vi "add scan current(SubVI).vi"(10 "字符串":string) -> (1 "ok or cancel":bool=TRUE, 2 "连接的字符串":string)   [LabVIEW 2019, in "SubVI.lvlib"]
uses:
  SubVI.lvlib
panel:
  in  "Number of Step":i32=2
  in  "Increments (mA)":dbl=10.0
  in  "Final Current (mA)":dbl
  in  "Initial Current(mA)":dbl
  in  "cancel":bool
  in  "ok":bool
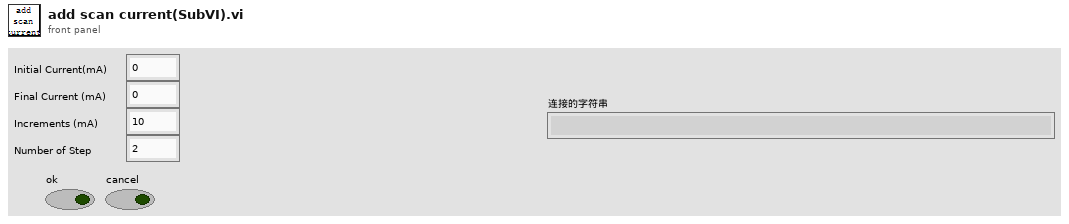
[diagram p1: front panel]
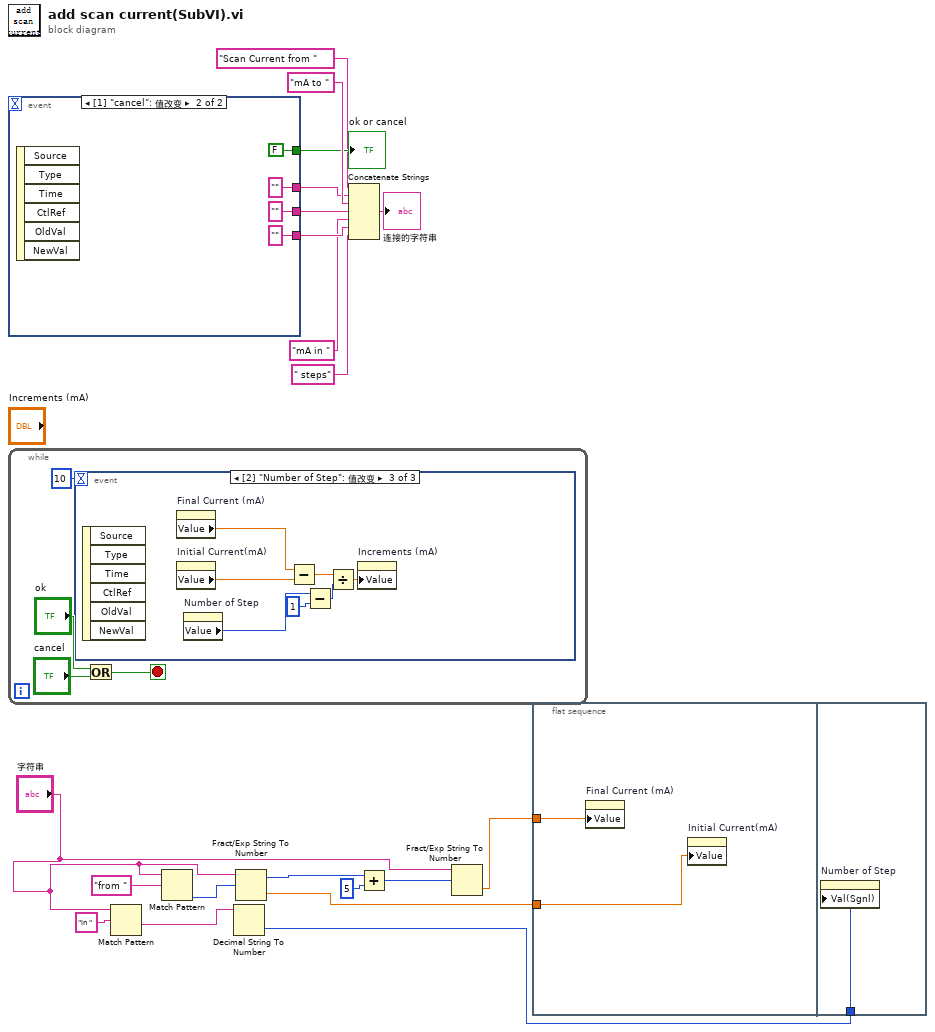
[diagram p0: block diagram]
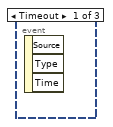
[diagram p2: hidden frame]
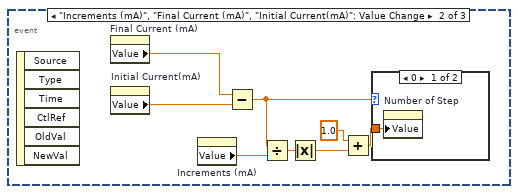
[diagram p3: hidden frame]
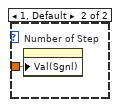
[diagram p4: hidden frame]
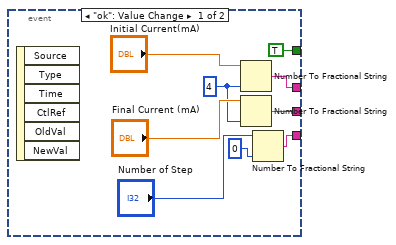
[diagram p5: hidden frame]
diagram:
  n1 = event shown="[1] \"cancel\": 值改变" {
    selector: _ -> [_ _]
    dyn-events: _ -> [_ _]
    timeout: _ -> [_ _]
    tunnel: [TRUE FALSE] -> w18
    tunnel: [w27 ""] -> w16
    tunnel: [w25 ""] -> w14
    tunnel: [w22 ""] -> w13
    event "ok": Value Change {
      w23 = i16 4 ("精度(6)")
      n2 = event-data() -> ()  [unwired: 1 in, 6 out]
      n3 = Number To Fractional String(number="Initial Current(mA)", precision (6)=w23) -> (F-format string=w27:string)  [unwired: 2 in]
      n4 = Number To Fractional String(number="Final Current (mA)", precision (6)=w23) -> (F-format string=w22:string)  [unwired: 2 in]
      n5 = Number To Fractional String(number="Number of Step", precision (6)=i16 0 ("精度(6)")) -> (F-format string=w25:string)  [unwired: 2 in]
    }
    event "cancel": Value Change {
      n6 = event-data() -> ()  [unwired: 1 in, 6 out]
    }
  }
  "ok or cancel" <- w18
  n7 = while {
    stop <- w36 stop-if-true
    n8 = event shown="[2] \"Number of Step\": 值改变" {
      selector: _ -> [_ _ _]
      dyn-events: _ -> [_ _ _]
      timeout: 10 -> [_ _ _]
      event Timeout {
        n9 = event-data() -> ()  [unwired: 1 in, 3 out]
      }
      event "Increments (mA)", "Final Current (mA)", "Initial Current(mA)": Value Change {
        n10 = event-data() -> ()  [unwired: 1 in, 6 out]
        n11 = property on="Final Current (mA)" class="DigNum (严格)"() -> ("Value"=w42:dbl)  [unwired: 2 in, 2 out]
        n12 = property on="Initial Current(mA)" class="DigNum (严格)"() -> ("Value"=w41:dbl)  [unwired: 2 in, 2 out]
        n13 = property on="Increments (mA)" class="DigNum (严格)"() -> ("Value"=w40:dbl)  [unwired: 2 in, 2 out]
        n14 = Subtract(x=w42, y=w41) -> (x-y=w38:dbl)
        n15 = Divide(x=w38, y=w40) -> (x/y=w44:dbl)
        n16 = Absolute Value(x=w44) -> (abs(x)=w43:dbl)
        n17 = Add(x=1.0, y=w43) -> (x+y=w39:dbl)
        n18 = case shown="0" w38 {
          tunnel: w39 -> [w46 w47]
          frame 0 {
            n19 = property on="Number of Step" class="DigNum (严格)"("Value"=w46) -> ()  [unwired: 2 in, 2 out]
          }
          frame 1, Default {
            n20 = property on="Number of Step" class="DigNum (严格)"("Val(Sgnl)"=w47) -> ()  [unwired: 2 in, 2 out]
          }
        }
      }
      event "Number of Step": Value Change {
        n21 = event-data() -> ()  [unwired: 1 in, 6 out]
        n22 = property on="Final Current (mA)" class="DigNum (严格)"() -> ("Value"=w51:dbl)  [unwired: 2 in, 2 out]
        n23 = property on="Initial Current(mA)" class="DigNum (严格)"() -> ("Value"=w50:dbl)  [unwired: 2 in, 2 out]
        n24 = property on="Number of Step" class="DigNum (严格)"() -> ("Value"=w49:i32)  [unwired: 2 in, 2 out]
        n25 = Subtract(x=w51, y=w50) -> (x-y=w54:dbl)
        n26 = Subtract(x=w49, y=1) -> (x-y=w52:i32)
        n27 = Divide(x=w54, y=w52) -> (x/y=w48:dbl)
        n28 = property on="Increments (mA)" class="DigNum (严格)"("Value"=w48) -> ()  [unwired: 2 in, 2 out]
      }
    }
    n29 = Or(x="ok", y="cancel") -> (x .or. y?=w36:bool)
  }
  n30 = Match Pattern(string="字符串", regular expression="in " ("正则表达式")) -> (after substring=w5:string)  [unwired: 1 in, 3 out]
  n31 = Match Pattern(string="字符串", regular expression="from " ("正则表达式")) -> (offset past match=w9:i32)  [unwired: 1 in, 3 out]
  n32 = Decimal String To Number(string=w5) -> (number=w1:i32)  [unwired: 2 in, 1 out]
  n33 = Fract/Exp String To Number(string="字符串", offset=w9) -> (offset past number=w7:i32, number=w3:dbl)  [unwired: 2 in]
  n34 = Concatenate Strings("Scan Current from " ("字符串"), w16, "mA to " ("字符串"), w13, "mA in " ("字符串"), w14, " steps" ("字符串")) -> (→"连接的字符串":string)
  n35 = Add(x=w7, y=5) -> (x+y=w8:i32)
  n36 = Fract/Exp String To Number(string="字符串", offset=w8) -> (number=w2:dbl)  [unwired: 2 in, 1 out]
  n37 = flat-sequence {
    tunnel: w3 -> [w56]
    tunnel: w2 -> [w55]
    tunnel: w1 -> [w57]
    frame #0 {
      n38 = property on="Final Current (mA)" class="DigNum (严格)"("Value"=w55) -> ()  [unwired: 2 in, 2 out]
      n39 = property on="Initial Current(mA)" class="DigNum (严格)"("Value"=w56) -> ()  [unwired: 2 in, 2 out]
    }
    frame #1 {
      n40 = property on="Number of Step" class="DigNum (严格)"("Val(Sgnl)"=w57) -> ()  [unwired: 2 in, 2 out]
    }
  }
